vi "h.SYSTEM.SetLaserScanSpeed.vi"(8 "error in":errorcluster, 10 "scan rate":u16=1000, 11 "Connection ID in":refnum<k5>) -> (0 "error out":errorcluster, 3 "Connection ID out":refnum<k5>)   [LabVIEW 2016, in "h.Library.lvlib"]
uses:
  h.Library.lvlib
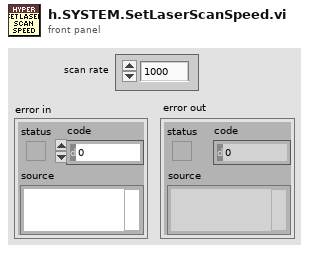
[diagram p1: front panel]
types:
  T1 = typedef "h.Library.lvlib/h.COMM.Command Status Enum.ctl" = enum8{"Success", "Failed", "Error", "AccessDenied", "InvalidCommand", "InvalidNumberArguments", "InvalidArgument", ""}
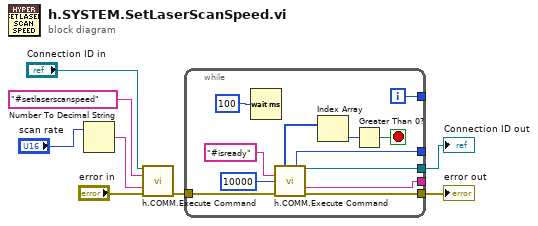
[diagram p0: block diagram]
diagram:
  n1 = Number To Decimal String(number="scan rate") -> (decimal integer string=w5:string)  [unwired: 1 in]
  n2 = call "h.COMM.Execute Command.vi"("Connection ID"="Connection ID in", "Command"="#setlaserscanspeed", "Argument"=w5, "error in"="error in") -> ("error out"=w3:errorcluster)  [unwired: 4 in, 7 out]
  n3 = while {
    tunnel: w3 -> [w15]
    tunnel: [w14] -> w2
    tunnel: [w13] -> w1
    tunnel: [w12] -> _
    tunnel: [w11] -> _
    tunnel: [w10] -> _
    i -> [w12]
    stop <- w17 stop-if-true
    n4 = Wait (ms)(milliseconds to wait=u32 100) -> ()  [unwired: 1 out]
    n5 = call "h.COMM.Execute Command.vi"("Command"="#isready", "Timeout"=10000, "error in"=w15) -> ("Content"=w19:u8[], "Status"=w11:T1, "Connection ID out"=w13:refnum<k5>, "Message"=w10:string, "error out"=w14:errorcluster)  [unwired: 5 in, 3 out]
    n6 = Index Array(array=w19) -> (element=w18:u8)  [unwired: 1 in]
    n7 = Greater Than 0?(x=w18) -> (x > 0?=w17:bool)
  }
  "error out" <- w2
  "Connection ID out" <- w1
